vi "Get Image Timings.vi"(8 "error in (no error)":errorcluster, 10 "Kinetic Series Lenght":u16, 11 "Header in":refnum<class "Header.lvclass">) -> (0 "error out":errorcluster, 2 "Base image name":string, 3 "Header out":refnum<class "Header.lvclass">)   [LabVIEW 2018, in "Header.lvclass"]
uses:
  Header.lvclass
  C:/Users/observer/Desktop/SPARC4_ACS/Simulated_Header/Simulated_Header.lvclass
  Simulated_Header/Simulated_Header.lvclass
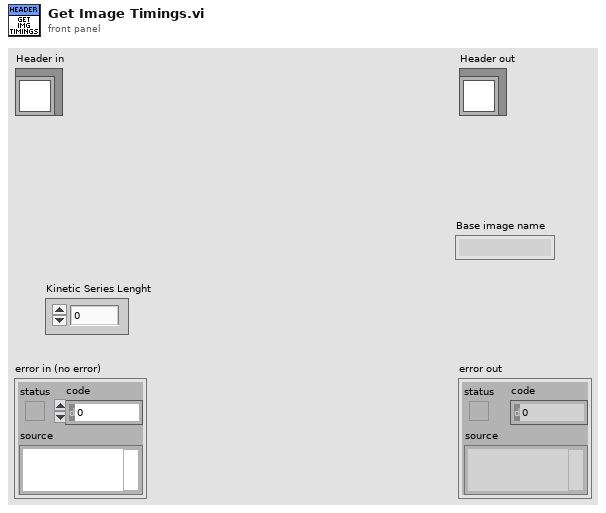
[diagram p1: front panel]
types:
  T1 = typedef "SYSTEMTIME structure typedef.ctl" = cluster{"Year":u16, "Month":u16, "DayOfWeek":u16, "Date":u16, "Hour":u16, "Minute":u16, "Second":u16, "Milliseconds":u16}
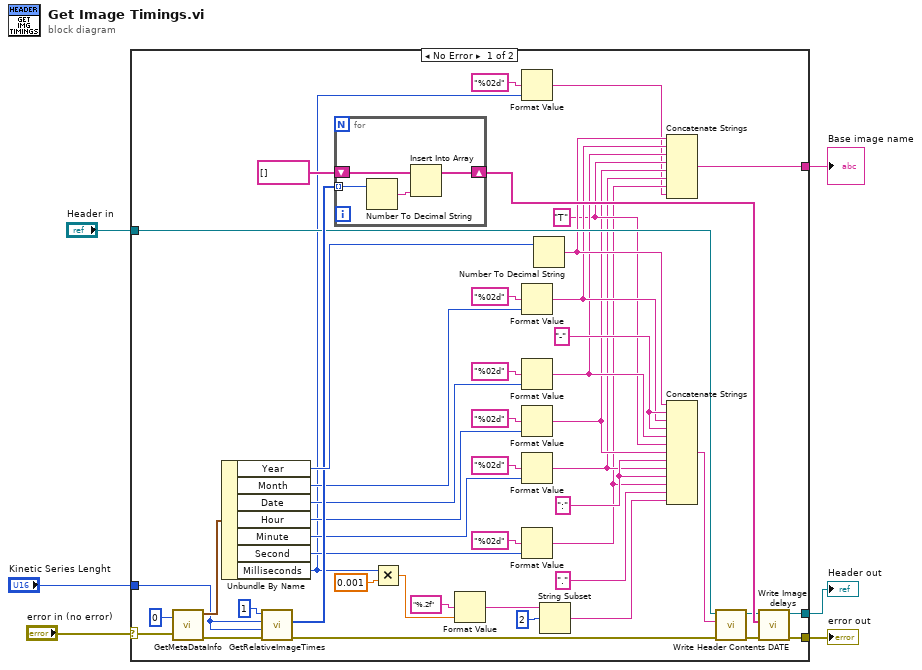
[diagram p0: block diagram]
diagram:
  n1 = case shown="No Error" "error in (no error)" {
    selector: "error in (no error)" -> [w27 w59]
    tunnel: [w18 w59] -> w2
    tunnel: [w21 w58] -> w3
    tunnel: "Header in" -> [w23 w58]
    tunnel: "Kinetic Series Lenght" -> [w26 _]
    tunnel: [w10 _] -> w1
    frame No Error {
      w47 = ":"
      w14 = "T"
      w48 = "-"
      n2 = call <userlib>:"GetMetaDataInfo.vi"("index"=0, "error in (no error)"=w27) -> ("SYSTEMTIME"=w53:T1, "error out"=w51:errorcluster)  [unwired: 2 out]
      n3 = Unbundle By Name(w53) -> ("Year"=w52:u16, "Month"=w38:u16, "Date"=w37:u16, "Hour"=w36:u16, "Minute"=w35:u16, "Second"=w34:u16, "Milliseconds"=w8:u16)
      n4 = call <userlib>:"GetRelativeImageTimes.vi"("error in (no error)"=w51, "size"=w26, "last"=w26, "first"=u32 1) -> ("error out"=w20:errorcluster, "arr"=w50:u64[])  [unwired: 5 in, 1 out]
      n5 = for {
        shift-right: [w54] -> w25
        shift-left: string[] [] -> [w55]
        tunnel: w50 -> [w57] mode=indexing
        n6 = Number To Decimal String(number=w57) -> (decimal integer string=w56:string)  [unwired: 1 in]
        n7 = Insert Into Array(array=w55, new element=w56) -> (w54:string[])  [unwired: 1 in]
      }
      n8 = Multiply(x=w8, y=0.001) -> (x*y=w33:dbl)
      n9 = Format Value(format string="%.2f", value (0)=w33) -> (output string=w32:string)  [unwired: 1 in]
      n10 = Format Value(format string="%02d", value (0)=w8) -> (output string=w7:string)  [unwired: 1 in]
      n11 = Format Value(format string="%02d", value (0)=w38) -> (output string=w16:string)  [unwired: 1 in]
      n12 = Format Value(format string="%02d", value (0)=w37) -> (output string=w15:string)  [unwired: 1 in]
      n13 = Format Value(format string="%02d", value (0)=w36) -> (output string=w13:string)  [unwired: 1 in]
      n14 = Format Value(format string="%02d", value (0)=w35) -> (output string=w12:string)  [unwired: 1 in]
      n15 = Format Value(format string="%02d", value (0)=w34) -> (output string=w11:string)  [unwired: 1 in]
      n16 = Number To Decimal String(number=w52) -> (decimal integer string=w17:string)  [unwired: 1 in]
      n17 = String Subset(string=w32, offset (0)=2) -> (substring=w28:string)  [unwired: 1 in]
      n18 = Concatenate Strings(w17, w16, w15, w14, w13, w12, w11, w7) -> (w10:string)
      n19 = Concatenate Strings(w17, w48, w16, w48, w15, w14, w13, w47, w12, w47, w11, ".", w28) -> (w24:string)
      n20 = call "Write Header Contents DATE.vi"("error in (no error)"=w20, "Header Content.DATE.Value"=w24, "Simulated_Header in"=w23) -> ("error out"=w19:errorcluster, "Simulated_Header out"=w22:refnum<class "Header.lvclass">)  [unwired: 7 in]
      n21 = call "Write Image delays.vi"("error in (no error)"=w19, "Image delays"=w25, "Header in"=w22) -> ("error out"=w18:errorcluster, "Header out"=w21:refnum<class "Header.lvclass">)  [unwired: 7 in]
    }
    frame Error {
    }
  }
  "error out" <- w2
  "Header out" <- w3
  "Base image name" <- w1
